vi "st_str Acquire Data from Hardware.vi"(8 "error in (no error)":errorcluster, 11 "Hardware Configuration":T1) -> (0 "error out":errorcluster, 1 "Array":cluster{dbl[], dbl[]}[](array[cluster]), 2 "Graph Data":waveform(dbl)[](array[waveform]))   [LabVIEW 2017]
doc: "Generates sample waveforms according to the signal type in the HW Config input."
uses:
  controls/st_str HW Configuration.ctl
  controls/st_str Simulated Signal Type.ctl
  <vilib>/Analysis/NI_AALBase.lvlib
panel:
  out "XY Graph":cluster{dbl[], dbl[]}(graph)
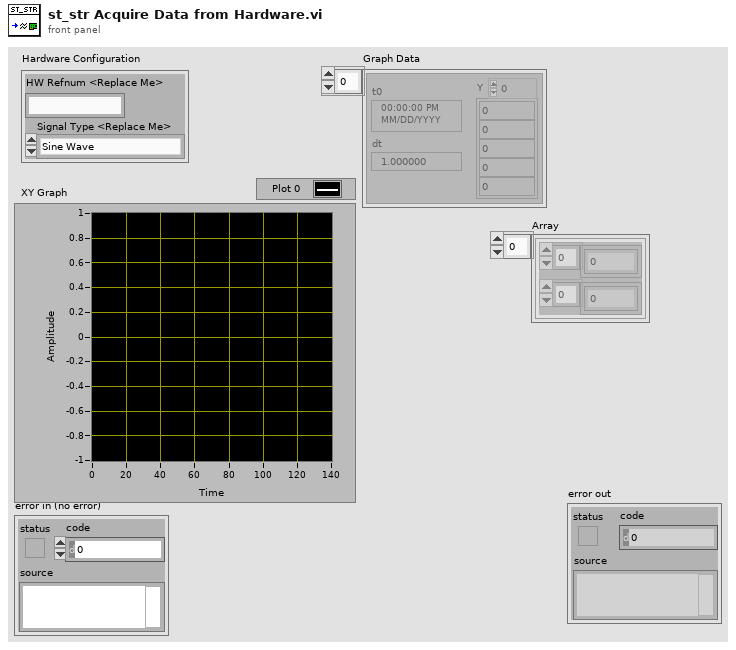
[diagram p1: front panel]
types:
  T1 = typedef "st_str HW Configuration.ctl" = cluster{"HW Refnum <Replace Me>":string, "Signal Type <Replace Me>":T2}
  T2 = typedef "st_str Simulated Signal Type.ctl" = enum16{"Sine Wave", "Square Wave"}
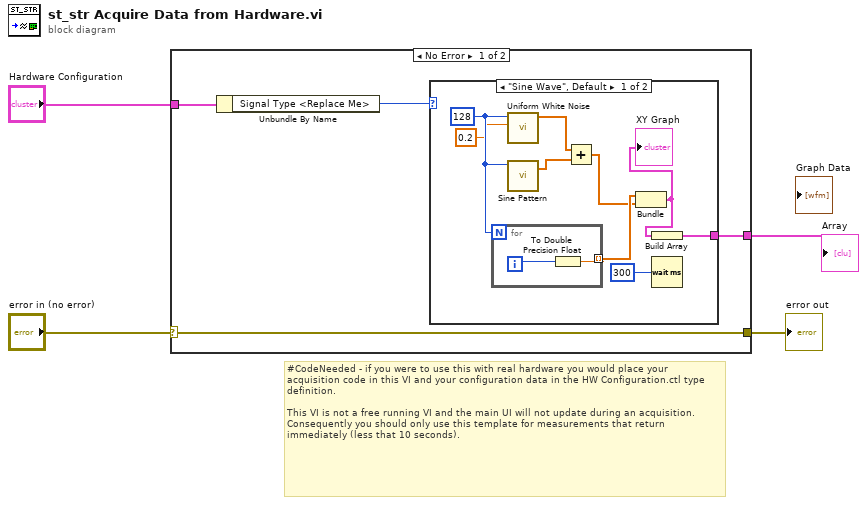
[diagram p0: block diagram]
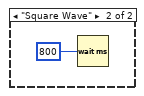
[diagram p2: hidden frame]
diagram:
  # "#CodeNeeded - if you were to use this with real hardware you would place your acquisition code in this VI and your configuration data in the HW Configuration.ctl type definition.\n\nThis VI is not a free running VI and the main UI will not update during an acquisition.  Consequently you should only use this template for measurements that return immediately (less that 10 seconds)."
  n1 = case shown="No Error" "error in (no error)" {
    selector: "error in (no error)" -> [w8 w21]
    tunnel: [w8 w21] -> w3
    tunnel: "Hardware Configuration" -> [w7 _]
    tunnel: [w5 _] -> w1
    frame No Error {
      n2 = Unbundle By Name(w7) -> ("Signal Type <Replace Me>"=w6:T2)
      n3 = case shown="\"Sine Wave\", Default" w6 {
        tunnel: [w11 _] -> w5
        frame "Sine Wave", Default {
          w17 = 128 ("samples")
          n4 = for {
            N: w17 -> [_]
            tunnel: [w18] -> w13 mode=indexing
            i -> [w19]
            n5 = To Double Precision Float(number=w19) -> (double precision float=w18:dbl)
          }
          n6 = call <vilib>:"Uniform White Noise.vi"("amplitude"=0.2, "samples"=w17) -> ("uniform white noise"=w15:dbl[])  [unwired: 8 in, 1 out]
          n7 = call <vilib>:"Sine Pattern.vi"("samples"=w17) -> ("Sinusoidal Pattern"=w14:dbl[])  [unwired: 3 in, 1 out]
          n8 = Add(x=w15, y=w14) -> (x+y=w12:dbl[])
          n9 = Bundle(w13, w12) -> (w10:cluster{dbl[], dbl[]})  [unwired: 1 in]
          "XY Graph" <- w10
          n10 = Build Array(w10) -> (w11:cluster{dbl[], dbl[]}[])
          n11 = Wait (ms)(milliseconds to wait=u32 300) -> ()  [unwired: 1 out]
        }
        frame "Square Wave" {
          n12 = Wait (ms)(milliseconds to wait=u32 800) -> ()  [unwired: 1 out]
        }
      }
    }
    frame Error {
    }
  }
  "error out" <- w3
  "Array" <- w1
